vi "Calculate Observables.vi"(7 "Analysis Framework":refnum<class "Analysis Framework.lvclass">, 8 "error in (no error)":errorcluster, 11 "Optimiser Cell in":refnum<class "Optimiser Cell.lvclass">) -> (0 "error out":errorcluster, 2 "Retry?":bool, 3 "Optimiser Cell out":refnum<class "Optimiser Cell.lvclass">)   [LabVIEW 2020, in "CIRCUS_uServices.lvlib" / "Run Utilities.lvlib" / "Optimiser Cell.lvclass"]
uses:
  Optimiser Cell.lvclass
  Analysis Framework/Analysis Framework.lvclass
  Optimiser Cell.lvclass/Optimiser Cell.ctl
  Optimiser Results.ctl
  Name with value pair.ctl
  TALOS/TALOS_PPL.lvlibp
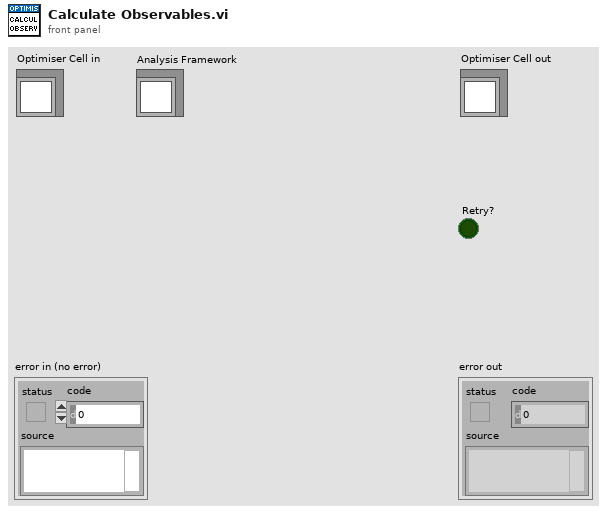
[diagram p1: front panel]
types:
  T1 = typedef "CIRCUS_uServices.lvlib/Run Utilities.lvlib/Optimiser Cell.lvclass/Optimiser Results.ctl" = cluster{"Array of Parameters":T2[], "Target":string}
  T2 = typedef "CIRCUS_uServices.lvlib/Analysis Framework.lvclass/Name with value pair.ctl" = cluster{"Name":string, "Value":string}
  T3 = typedef "CIRCUS_uServices.lvlib/Run Utilities.lvlib/Optimiser Cell.lvclass/Optimisation observable.ctl" = cluster{"Name":string, "Weight":dbl}
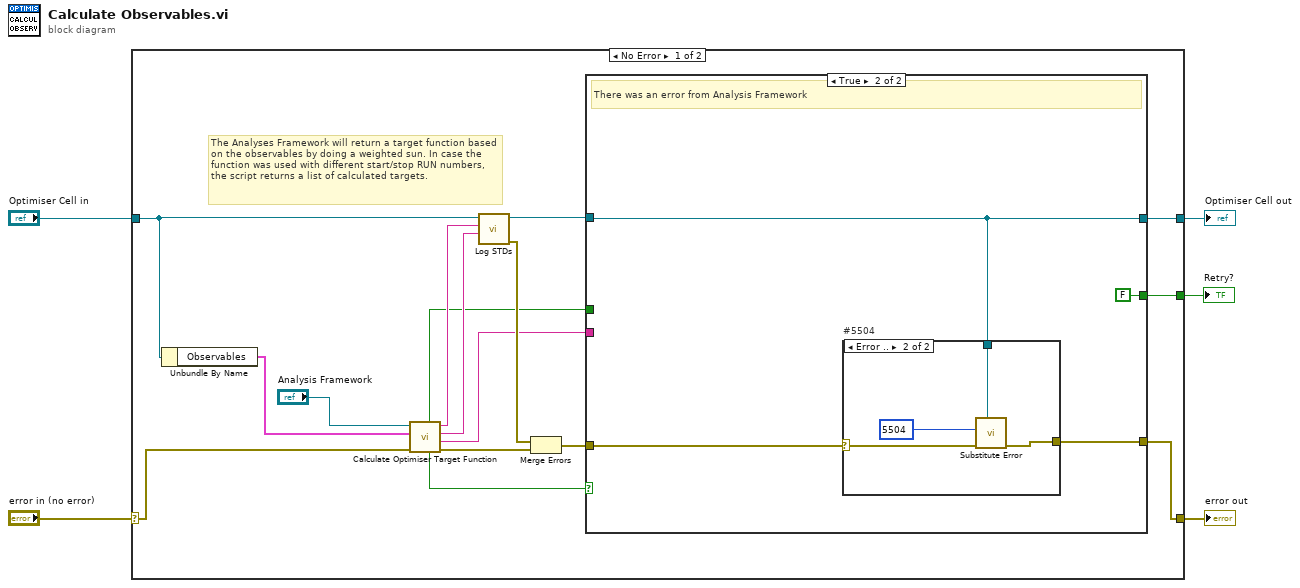
[diagram p0: block diagram]
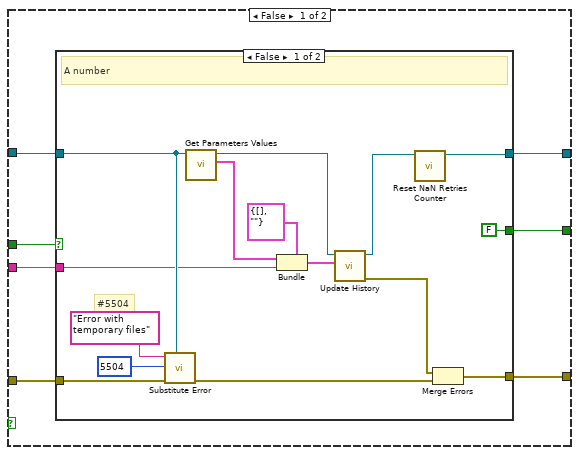
[diagram p2: hidden frame]
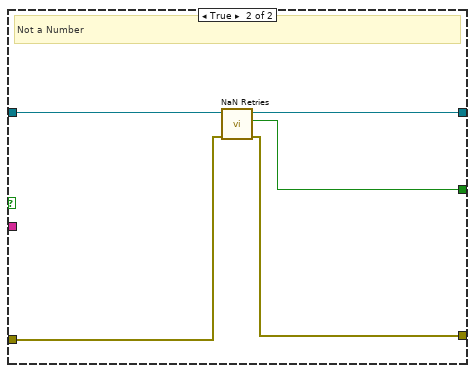
[diagram p3: hidden frame]
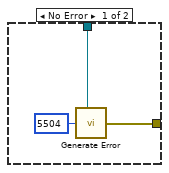
[diagram p4: hidden frame]
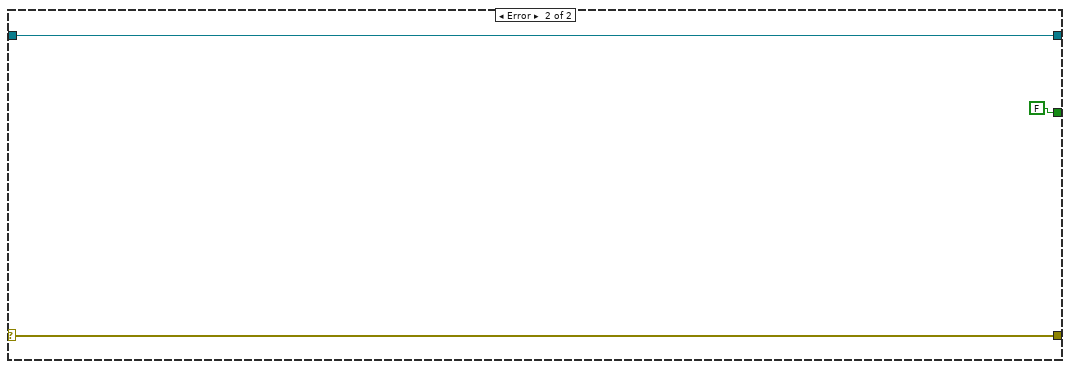
[diagram p5: hidden frame]
diagram:
  n1 = case shown="No Error" "error in (no error)" {
    selector: "error in (no error)" -> [w16 w62]
    tunnel: [w20 w62] -> w4
    tunnel: [w21 w61] -> w2
    tunnel: "Optimiser Cell in" -> [w13 w61]
    tunnel: [w6 FALSE ("Retry?")] -> w1
    frame No Error {
      # "The Analyses Framework will return a target function based on the observables by doing a weighted sun. In case the function was used with different start/stop RUN numbers, the script returns a list of calculated targets."
      n2 = Unbundle By Name(w13) -> ("Observables"=w18:T3[])
      n3 = call-dynamic "Calculate Optimiser Target Function.vi"("error in (no error)"=w16, "Observables"=w18, "Analysis Framework"="Analysis Framework") -> ("error out (no error)"=w15:errorcluster, "Target"=w8:string, "standard error"=w10:string, "standard output"=w11:string, "Error"=w14:bool, "NaN"=w7:bool)  [unwired: 3 in]
      n4 = call-dynamic "Log STDs.vi"("StdErr"=w10, "StdOut"=w11, "Run Optimiser in"=w13) -> ("error out"=w9:errorcluster, "Run Optimiser out"=w12:refnum<class "Optimiser Cell.lvclass">)  [unwired: 7 in]
      n5 = Merge Errors(w9, w15) -> (w19:errorcluster)
      n6 = case shown="True" w14 {
        tunnel: w8 -> [w24 _]
        tunnel: w12 -> [w25 w52]
        tunnel: [w28 w52] -> w21
        tunnel: [w27 w51] -> w20
        tunnel: w19 -> [w26 w50]
        tunnel: w7 -> [w23 _]
        tunnel: [w22 FALSE ("Retry?")] -> w6
        frame False {
          n7 = case shown="False" w23 {
            tunnel: [w29 w45] -> w28
            tunnel: [w43 w46] -> w27
            tunnel: w26 -> [w41 w47]
            tunnel: w25 -> [w37 w48]
            tunnel: w24 -> [w34 _]
            tunnel: [FALSE ("Retry?") w44] -> w22
            frame False {
              # "#5504"
              # "A number"
              n8 = call "Substitute Error.vi"("LabVIEW Object"=w37, "error in (no error)"=w41, "Error Code"=5504, "Optional String"="Error with temporary files") -> ("error out"=w40:errorcluster)  [unwired: 7 in]
              n9 = call-dynamic "Get Parameters Values.vi"("Run Optimiser in"=w37) -> ("Optimisation Parameters"=w35:T2[], "Run Optimiser out"=w36:refnum<class "Optimiser Cell.lvclass">)  [unwired: 8 in, 1 out]
              n10 = Bundle(cluster=T1 {"Array of Parameters"=[], "Target"=""} ("Optimisation result"), "Array of Parameters"=w35, "Target"=w34) -> (w31:T1)
              n11 = call-dynamic "Update History.vi"("Optimisation result"=w31, "Run Optimiser in"=w36) -> ("error out"=w42:errorcluster, "Run Optimiser out"=w30:refnum<class "Optimiser Cell.lvclass">)  [unwired: 8 in]
              n12 = call-dynamic "Reset NaN Retries Counter.vi"("Run Optimiser in"=w30) -> ("Run Optimiser out"=w29:refnum<class "Optimiser Cell.lvclass">)  [unwired: 9 in, 1 out]
              n13 = Merge Errors(w42, w40) -> (w43:errorcluster)
            }
            frame True {
              # "Not a Number"
              n14 = call-dynamic "NaN Retries.vi"("error in (no error)"=w47, "Optimiser Cell in"=w48) -> ("error out"=w46:errorcluster, "Retry?"=w44:bool, "Optimiser Cell out"=w45:refnum<class "Optimiser Cell.lvclass">)  [unwired: 7 in]
            }
          }
        }
        frame True {
          # "There was an error from Analysis Framework"
          n15 = case "#5504" shown="Error .." w50 {
            selector: w50 -> [_ w56]
            tunnel: w52 -> [w55 w59]
            tunnel: [w54 w58] -> w51
            frame No Error {
              n16 = call "Generate Error.vi"("Class"=w55, "Error Code"=5504) -> ("error out"=w54:errorcluster)  [unwired: 5 in]
            }
            frame Error {
              n17 = call "Substitute Error.vi"("LabVIEW Object"=w59, "error in (no error)"=w56, "Error Code"=5504) -> ("error out"=w58:errorcluster)  [unwired: 8 in]
            }
          }
        }
      }
    }
    frame Error {
    }
  }
  "error out" <- w4
  "Optimiser Cell out" <- w2
  "Retry?" <- w1
